vi "test NtripClient-2.vi"() -> ()   [LabVIEW 2019]
uses:
  Ctrl/Ntrip_Account_db.ctl
panel:
  out "에러 출력 2":errorcluster caption="에러 출력"
  in  "탭 컨트롤":enum32{"Main", "ref", "wireshark capture"}(tab)
  in  "Mount points":u16(ring) items=["FKP_V31", "SSRG", "VRS_V31", "VRS_V32"]
  out "RTCM recv":string
  in  "stop":bool
  in  "write":bool
  out "station\nconn":bool
  out "server name":string
  out "mount points":string[](array[string])
  out "연결된 문자열":string
  out "링 텍스트.텍스트":string
  out "n1":i32
  in  "Current Ntrip account":T1={"address"="gnss.eseoul.go.kr", "port "=2101, "id"="seoul", "pwd"="seoul", "ref pt"="YONS-RTCM32-M5"}
  in  "read bytes":i32=10000
  out "에러 출력":errorcluster
  out "데이터 출력":string
  # "fkp.ngii.go.kr"
  # "Test Ntrip Client"
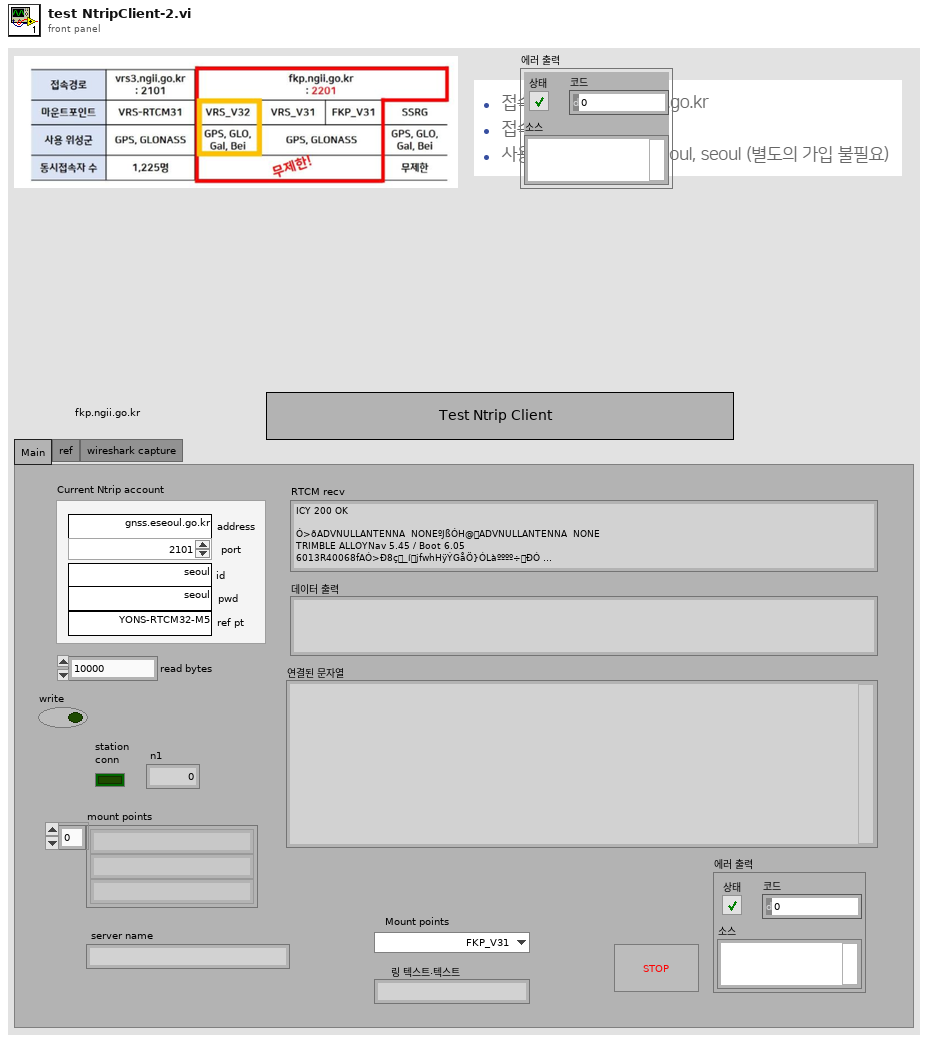
[diagram p1: front panel]
types:
  T1 = typedef "Ntrip_Account_db.ctl" = cluster{"address":string, "port ":u16, "id":string, "pwd":string, "ref pt":string}
  T2 = enum16{"Standard", "Buffered", "CRLF", "Immediate"}
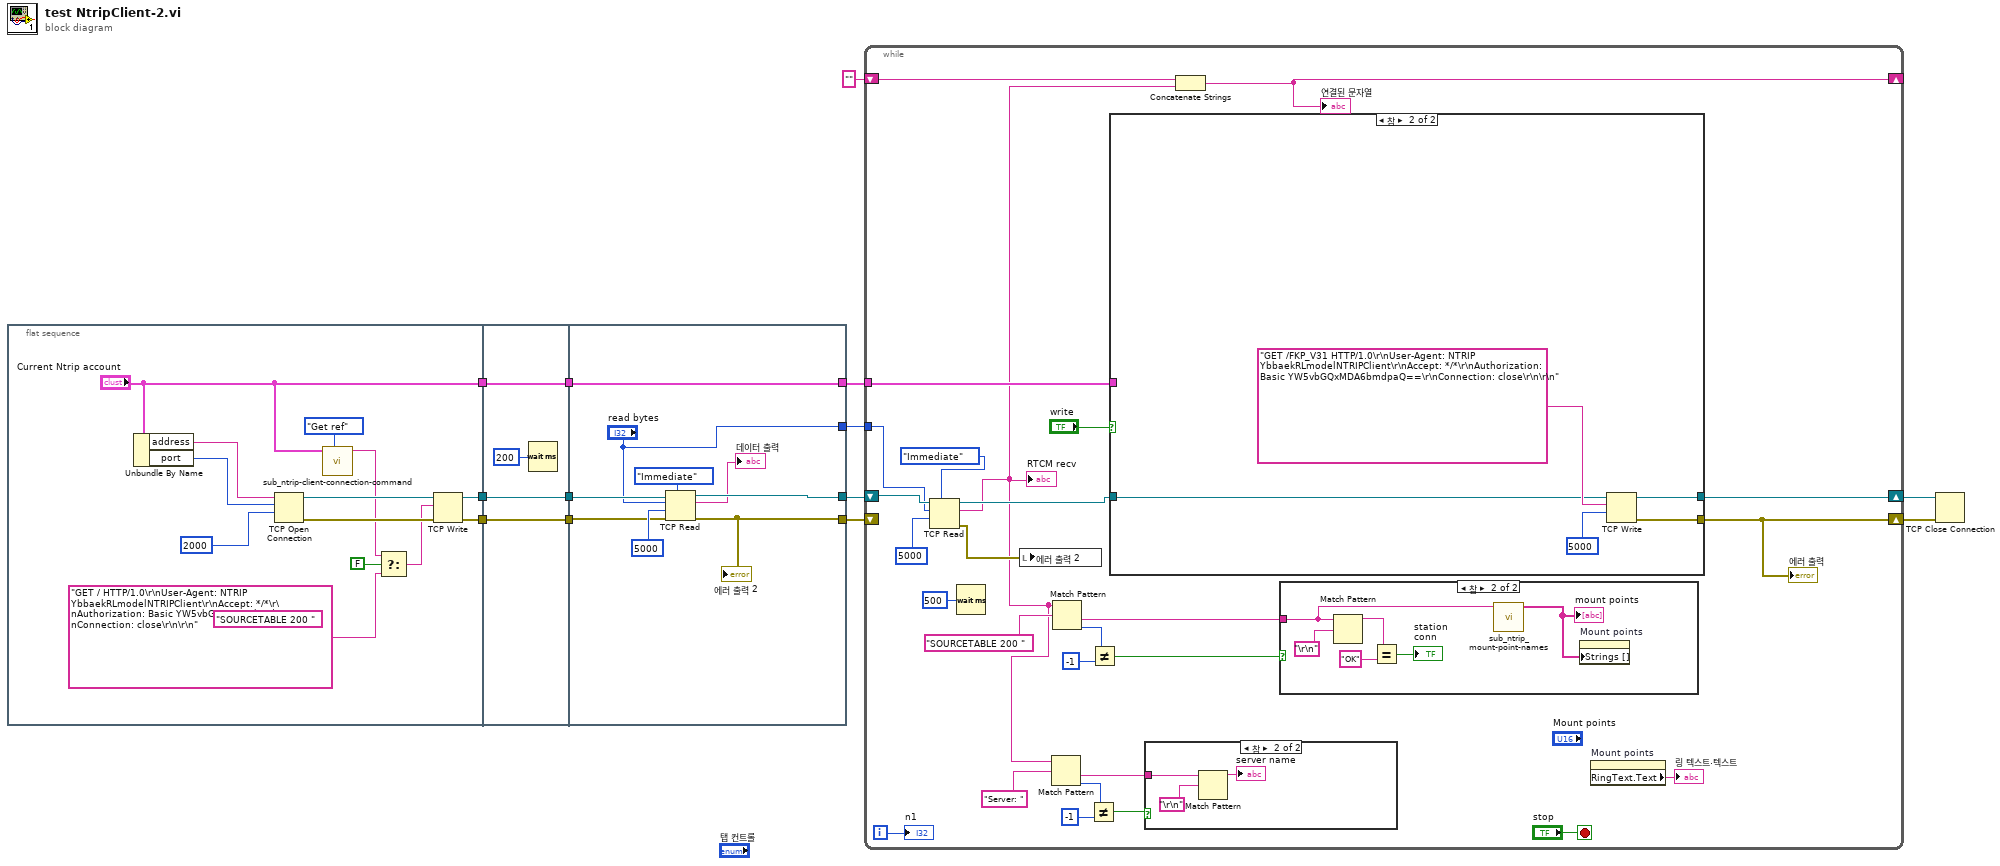
[diagram p0: block diagram]
diagram:
  n1 = flat-sequence {
    tunnel: [w24] -> w8
    tunnel: [w23] -> w7
    tunnel: ["Current Ntrip account"] -> w5
    tunnel: w8 -> [w30]
    tunnel: w7 -> [w29]
    tunnel: w5 -> [w27]
    tunnel: [w30] -> w4
    tunnel: [w29] -> w3
    tunnel: [w27] -> w2
    tunnel: [w39] -> w6
    tunnel: [w36] -> w10
    tunnel: [w32] -> w11
    tunnel: w4 -> [w34]
    tunnel: w3 -> [w35]
    tunnel: w2 -> [w39]
    tunnel: ["read bytes"] -> w1
    frame #0 {
      (unwired) "SOURCETABLE 200 " ("정규식")
      n2 = Unbundle By Name("Current Ntrip account") -> ("address"=w20:string, "port"=w19:u16)
      n3 = TCP Open Connection(address=w20, remote port or service name=w19, timeout ms (60000)=2000) -> (connection ID=w25:refnum<k5>, error out=w22:errorcluster)  [unwired: 2 in]
      n4 = call "sub_ntrip-client-connection-command.vi"("cmd"=enum16{"Get ref", "Get rtcm"}."Get ref", "Current Ntrip account"="Current Ntrip account") -> ("hex"=w16:string)  [unwired: 9 in]
      n5 = Select(t=w16, s=FALSE, f="GET / HTTP/1.0\r\nUser-Agent: NTRIP YbbaekRLmodelNTRIPClient\r\nAccept: */*\r\nAuthorization: Basic YW5vbGQxMDA6bmdpaQ==\r\nConnection: close\r\n\r\n" ("ascii 2")) -> (s? t:f=w14:string)
      n6 = TCP Write(connection ID=w25, data in=w14, error in (no error)=w22) -> (connection ID out=w23:refnum<k5>, error out=w24:errorcluster)  [unwired: 1 in, 1 out]
    }
    frame #1 {
      n7 = Wait (ms)(milliseconds to wait=u32 200) -> ()  [unwired: 1 out]
    }
    frame #2 {
      n8 = TCP Read(connection ID=w35, bytes to read="read bytes", error in (no error)=w34, 7:T2."Immediate" ("mode (standard)"), 9:5000 ("타임아웃 ms (25000)")) -> (connection ID out=w36:refnum<k5>, data out=→"데이터 출력":string, error out=w32:errorcluster)
      "에러 출력 2" <- w32
    }
  }
  n9 = while {
    shift-right: [w47] -> w12
    shift-left: w11 -> [_]
    shift-right: [w64] -> w13
    shift-left: w10 -> [w45]
    shift-right: [w51] -> _
    shift-left: "" -> [w62]
    tunnel: w6 -> [w48]
    tunnel: w1 -> [w40]
    i -> [w49]
    stop <- "stop" stop-if-true
    n10 = TCP Read(connection ID=w45, bytes to read=w40, 7:T2."Immediate" ("mode (standard)"), 9:5000 ("타임아웃 ms (25000)")) -> (connection ID out=w44:refnum<k5>, data out=w42:string, error out=w43:errorcluster)  [unwired: 1 in]
    "RTCM recv" <- w42
    n11 = Wait (ms)(milliseconds to wait=u32 500) -> ()  [unwired: 1 out]
    n12 = local write "에러 출력 2"(w43) -> ()
    n13 = Match Pattern(string=w42, regular expression="Server: " ("정규식")) -> (after substring=w53:string, offset past match=w55:i32)  [unwired: 1 in, 2 out]
    n14 = Match Pattern(string=w42, regular expression="SOURCETABLE 200 " ("정규식")) -> (after substring=w60:string, offset past match=w58:i32)  [unwired: 1 in, 2 out]
    n15 = Not Equal?(x=w55, y=-1) -> (x != y?=w56:bool)
    n16 = Not Equal?(x=w58, y=-1) -> (x != y?=w57:bool)
    n17 = case shown="참" "write" {
      tunnel: w44 -> [w76 w77]
      tunnel: [_ w81] -> w47
      tunnel: [w76 w80] -> w64
      tunnel: w48 -> [_ _]
      frame False {
      }
      frame True {
        n18 = TCP Write(connection ID=w77, data in="GET /FKP_V31 HTTP/1.0\r\nUser-Agent: NTRIP YbbaekRLmodelNTRIPClient\r\nAccept: */*\r\nAuthorization: Basic YW5vbGQxMDA6bmdpaQ==\r\nConnection: close\r\n\r\n" ("ascii 2"), 9:5000 ("타임아웃 ms (25000)")) -> (connection ID out=w80:refnum<k5>, error out=w81:errorcluster)  [unwired: 1 in, 1 out]
      }
    }
    "에러 출력" <- w47
    n19 = case shown="참" w56 {
      tunnel: w53 -> [_ w68]
      frame False {
      }
      frame True {
        n20 = Match Pattern(string=w68, regular expression="\r\n") -> (before substring=→"server name":string)  [unwired: 1 in, 3 out]
      }
    }
    n21 = Concatenate Strings(w62, w42) -> (w51:string)
    "연결된 문자열" <- w51
    n22 = case shown="참" w57 {
      tunnel: w60 -> [_ w71]
      frame False {
      }
      frame True {
        n23 = Match Pattern(string=w71, regular expression="\r\n") -> (before substring=w74:string)  [unwired: 1 in, 3 out]
        n24 = Equal?(x=w74, y="OK") -> (x = y?=→"station\nconn":bool)
        n25 = call "sub_ntrip_mount-point-names.vi"("ntrip str"=w71) -> ("mount points"=w70:string[])  [unwired: 10 in]
        "mount points" <- w70
        n26 = property on="Mount points" class="Ring (엄격한)"("Strings []"=w70) -> ()  [unwired: 2 in, 2 out]
      }
    }
    n27 = property on="Mount points" class="Ring (엄격한)"() -> ("RingText.Text"=→"링 텍스트.텍스트":string)  [unwired: 2 in, 2 out]
    "n1" <- w49
  }
  n28 = TCP Close Connection(connection ID=w13, error in (no error)=w12) -> ()  [unwired: 1 in, 2 out]
